vi "Measurement UI.vi"() -> ()   [LabVIEW 2021, in "Crosstalk_Audio ADC_UI.lvlib"]
uses:
  Crosstalk_Audio ADC_UI.lvlib
  shared/controls/PCM Interface Type_Copy.ctl
  <vilib>/PDM Acquisition Toolkit/shared/controls/Digital Edge.ctl
  shared/Audio ADC Shared.lvlib
  <vilib>/PDM Acquisition Toolkit/shared/PDM Shared.lvlib
  shared/controls/Audio ADC Controls.lvlib
panel:
  out "MeasTable":string[][](table)
  in  "MeasGraphs":T1(tab)=enum."Time Domain"
  out "FreqDomainGraph":cluster{"f0":dbl, "df":dbl, "Spectrum":dbl[]}[](graph) caption="AC"
  out "TimeDomainGraph":waveform(dbl)[](graph) caption="AC"
  out "Victim time domain":dbl[](array[numeric])
  out "Victim spectrum":dbl[](array[numeric])
  out "dt":dbl
  out "t0":dbl
  out "df":dbl
  out "f0":dbl
  out "Time domain":dbl[](array[numeric])
  out "Spectrum":dbl[](array[numeric])
  out "Crosstalk":dbl
  out "Channel":string
  in  "Victim channel resource name":string
  in  "Digital capture resource name":string
  in  "Configuration tab":enum32{"Protocol", "Measurement"}(tab)=enum."Measurement"
  in  "Endianness":enum32{"MSB First", "LSB First"}(ring)
  in  "Bit clock edge  sync":enum32{"Rising", "Falling"}(ring)=enum."Falling"
  in  "Frame sync edge for Channel 0":enum32{"Rising", "Falling"}(ring)=enum."Falling"
  in  "Channel count per frame":u32=2
  in  "Channel length":u32=32
  in  "Bit depth":u32=24
  in  "Channel 0 offset":u32=1
  in  "Data Justification":enum32{"Left Justified", "Right Justified"}(ring) caption="Data justification"
  in  "Frame length":u32=64
  in  "Frame sync pulse width":u32=32
  in  "I2S":bool
  in  "LJ":bool
  in  "RJ":bool
  in  "TDM":bool
  in  "Measurement Duration":dbl=0.1 caption="Measurement duration" format="%#_6ps"
  in  "Protocol capture resource name":string(combo) caption="Resource name"
  in  "Analog source resource name":string(combo) caption="Resource name"
  in  "Channel name":string
  in  "Full scale range":dbl=2.825 caption="FULL SCALE RANGE" format="%.3pV"
  in  "Data line":u32
  in  "Sample rate":dbl=192000.0 format="%#.6pHz"
  in  "Measurement settings":string="Measurement Settings"
  in  "Amplitude":dbl=-1.0 format="%#_6pdB"
  in  "Frequency":dbl=1000.0 format="%#_6pHz"
  in  "Victim channel":u32=1
  in  "Interferer channel":u32
  in  "Analog source":string="Analog source"
  in  "Digital capture":string="Digital capture"
  # "Protocols"
  # "PCM data configuration"
  # "Frame sync clock control"
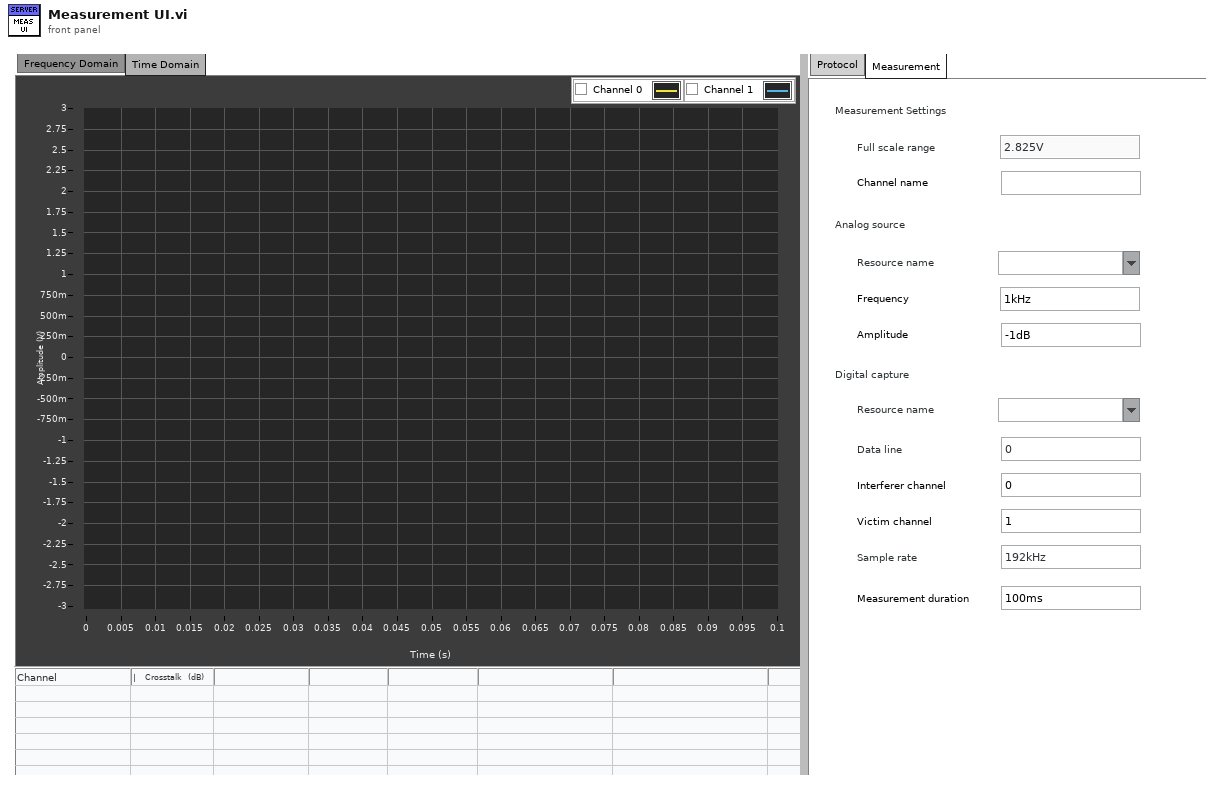
[diagram p1: front panel]
types:
  T1 = enum32{"Frequency Domain", "Time Domain", "Hidden Controls"}
  T2 = typedef "PDM Shared.lvlib/Digital Edge.ctl" = enum8{"Rising", "Falling"}
  T3 = typedef "Audio ADC Controls.lvlib/PCM Interface Type_Copy.ctl" = enum16{"I2S", "Left Justified", "Right Justified", "TDM 4 Channel", "TDM 6 Channel", "TDM 8 Channel", "DSP mode", "DSP mode with 1 bit delay", "PCM Short Frame", "PCM Long Frame"}
  T4 = typedef "PDM Shared.lvlib/PCM Frame Sync Control.ctl" = cluster{"Frame Length":u16, "Frame Sync Pulse Width":u16, "Bit Clock Edge  Sync":T2}
  T5 = typedef "PDM Shared.lvlib/PCM Data Format Configuration.ctl" = cluster{"Frame Sync Edge for Channel 0":T2, "Channel Count Per Frame":u8, "Channel Length":u16, "Bit Depth":u8, "Channel 0 Offset":u16, "Endianness":T6, "Data Justification":T7}
  T6 = typedef "PDM Shared.lvlib/PCM Bit Endianness.ctl" = enum16{"MSB First", "LSB First"}
  T7 = typedef "PDM Shared.lvlib/PCM Data Justification.ctl" = enum16{"Left Justified", "Right Justified"}
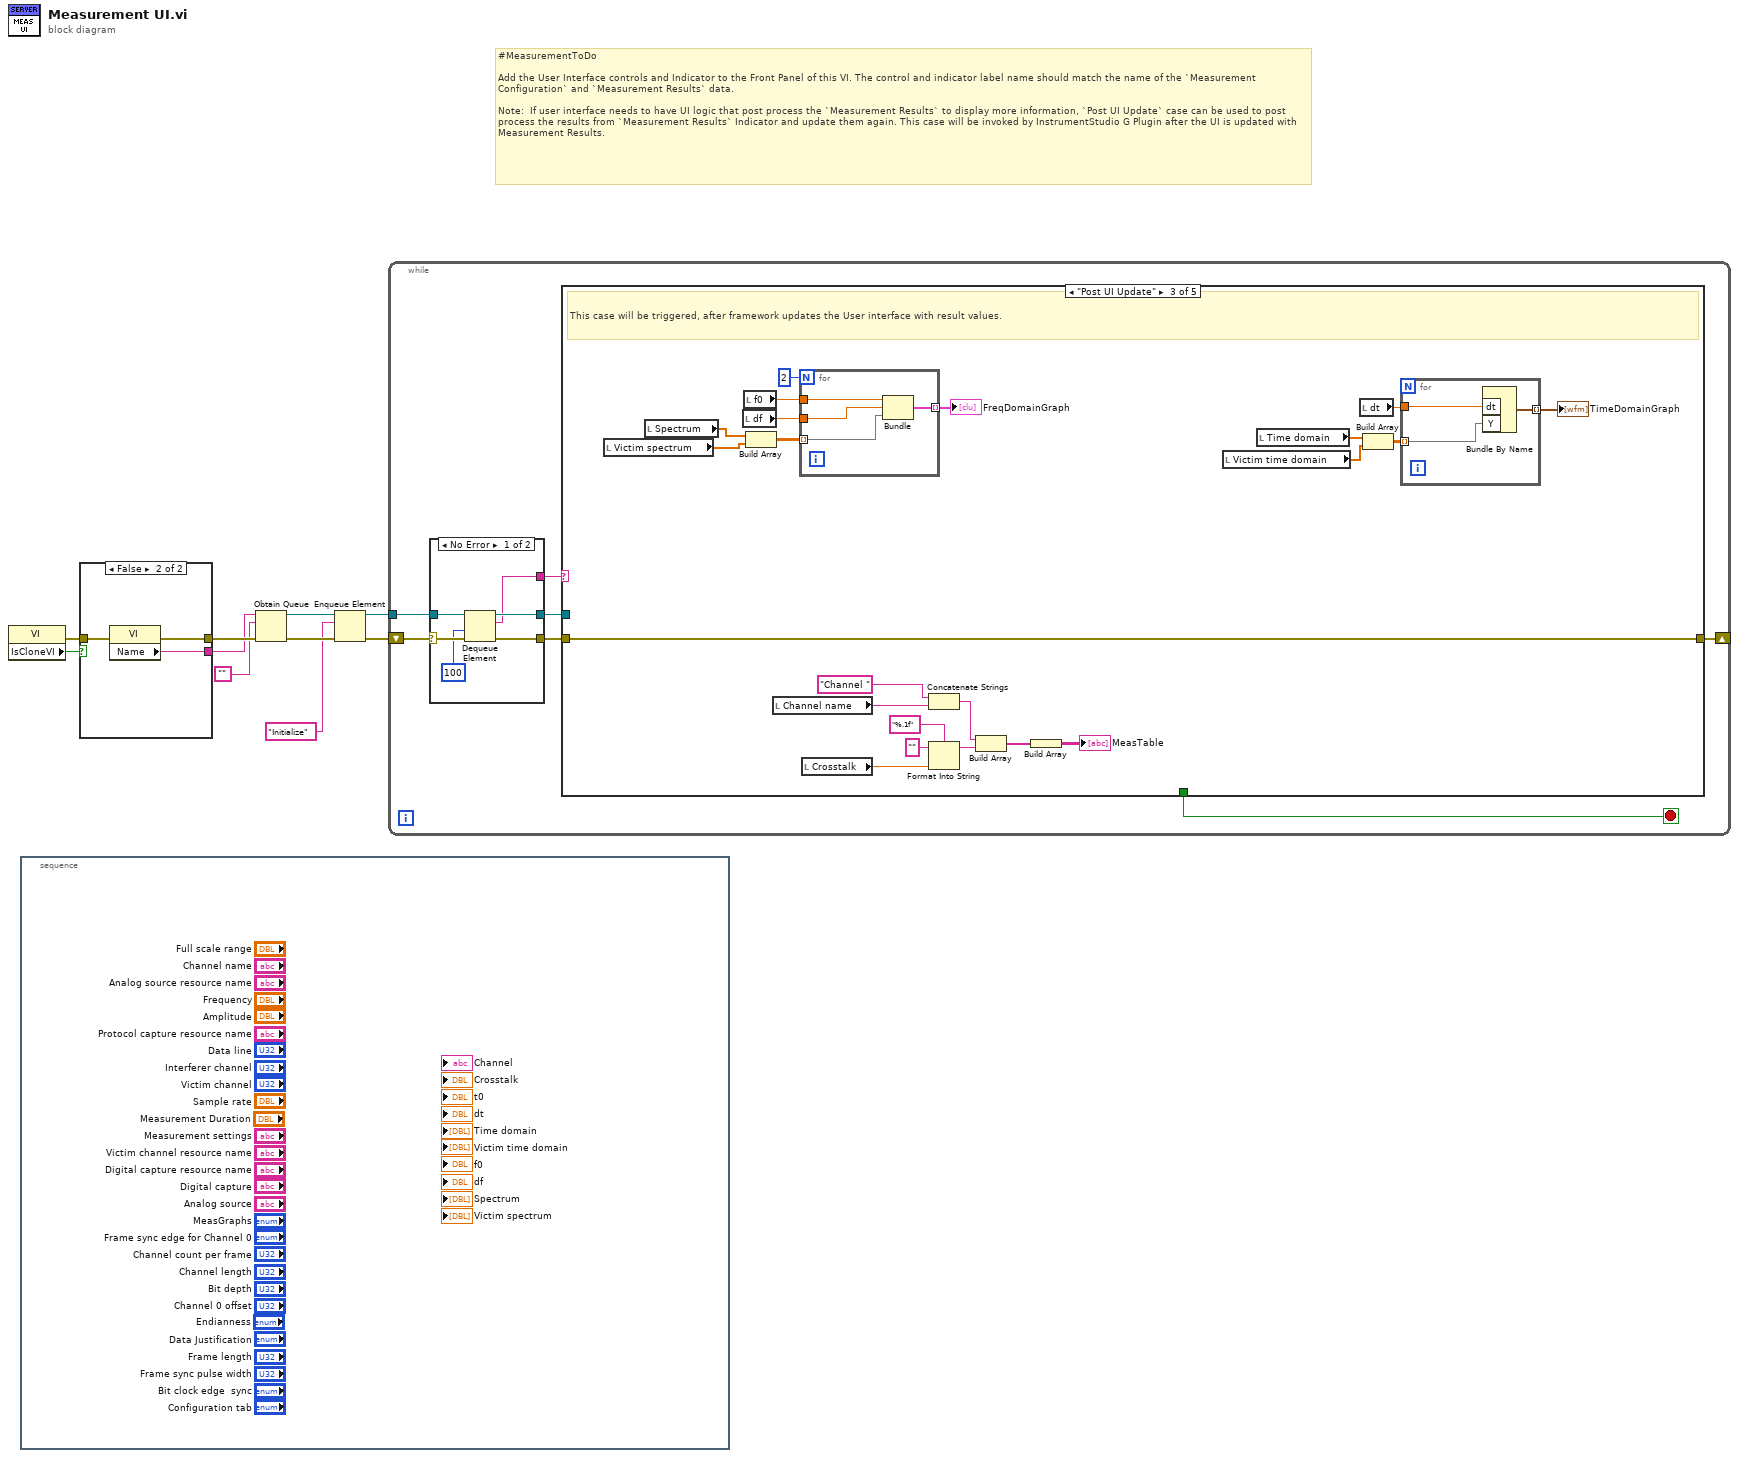
[diagram p0: block diagram]
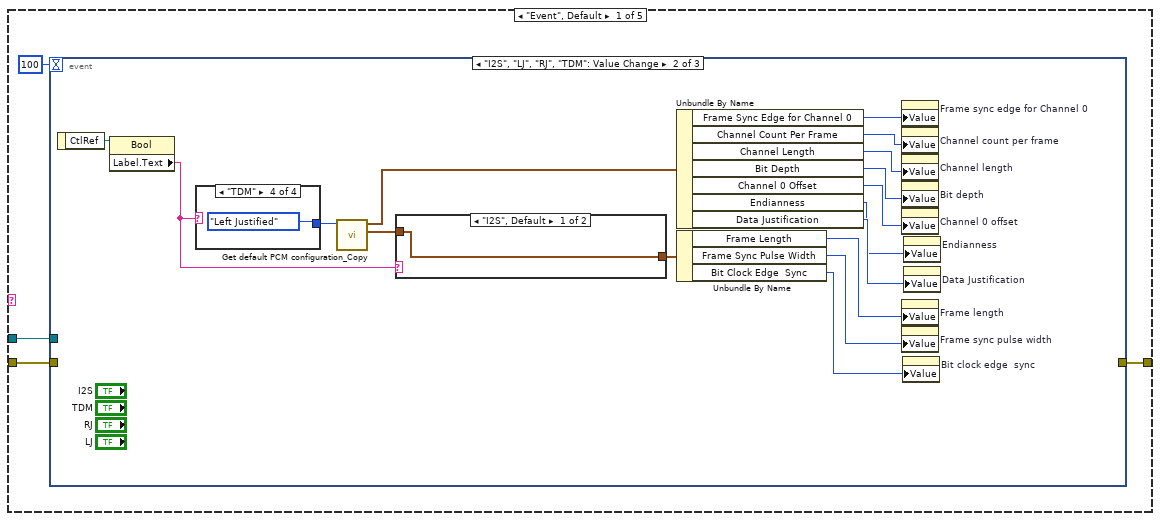
[diagram p2: hidden frame]
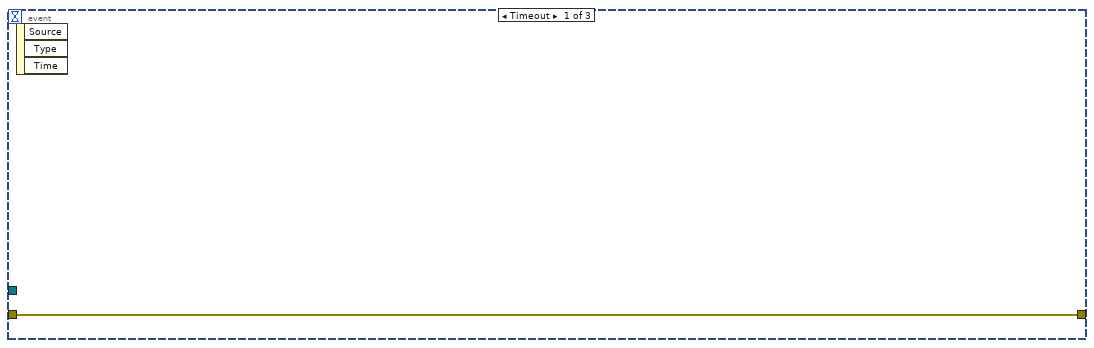
[diagram p3: hidden frame]
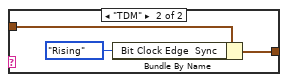
[diagram p4: hidden frame]
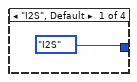
[diagram p5: hidden frame]
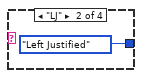
[diagram p6: hidden frame]
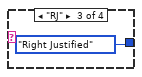
[diagram p7: hidden frame]
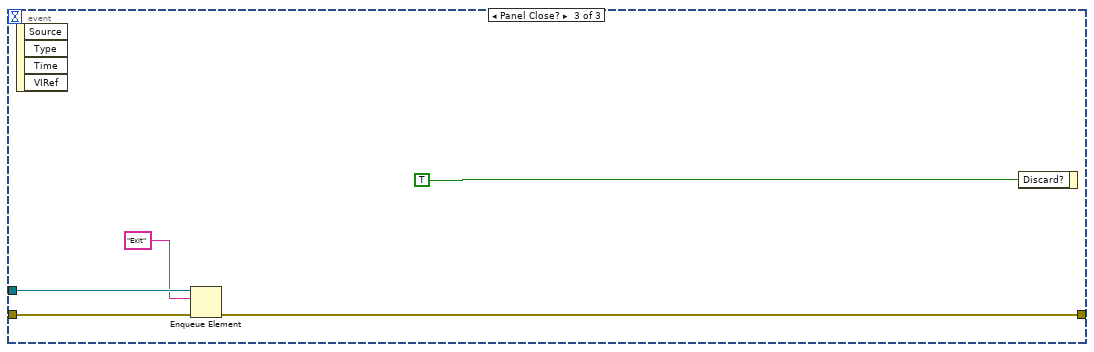
[diagram p8: hidden frame]
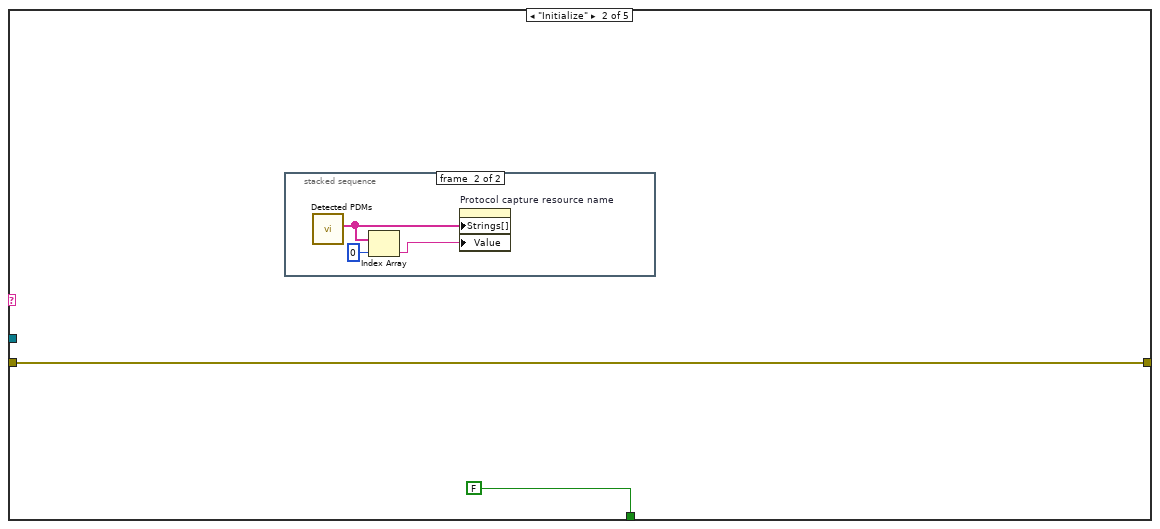
[diagram p9: hidden frame]
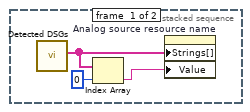
[diagram p10: hidden frame]
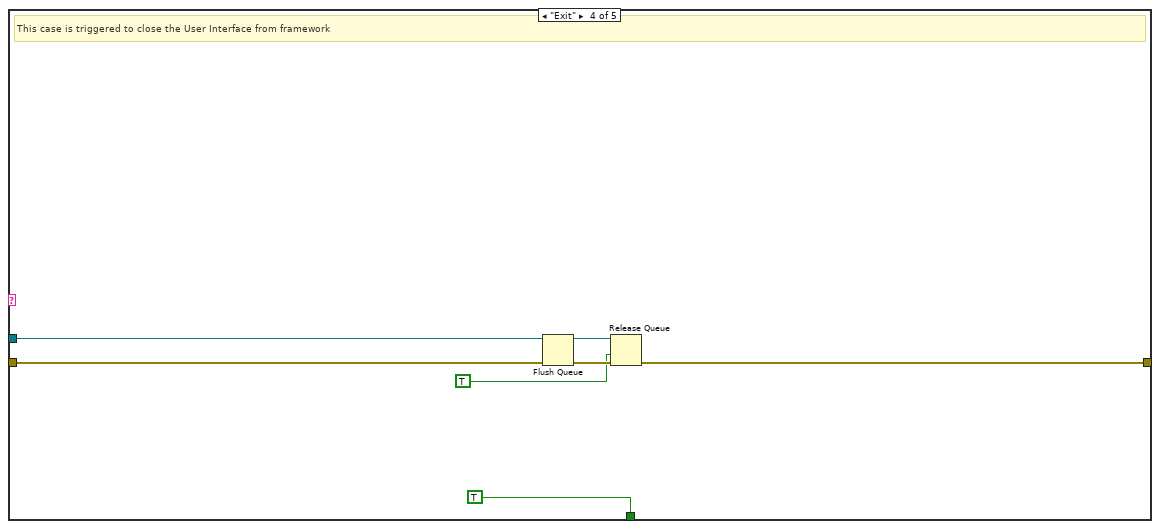
[diagram p11: hidden frame]
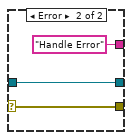
[diagram p13: hidden frame]
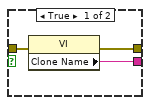
[diagram p14: hidden frame]
diagram:
  # "#MeasurementToDo  \n\nAdd the User Interface controls and Indicator to the Front Panel of this VI. The control and indicator label name should match the name of the `Measurement Configuration` and `Measurement Results` data.\n\nNote:  If user interface needs to have UI logic that post process the `Measurement Results` to display more information, `Post UI Update` case can be used to post process the results from `Measurement Results` Indicator and update them again. This case will be invoked by InstrumentStudio G Plugin after the UI is updated with Measurement Results."
  n1 = property class="VI"() -> (error out=w1:errorcluster, "IsCloneVI"=w2:bool)  [unwired: 2 in, 1 out]
  n2 = stacked-sequence {
    frame #0 {
    }
  }
  n3 = case shown="False" w2 {
    tunnel: [w13 w16] -> w10
    tunnel: [w12 w15] -> w9
    tunnel: w1 -> [w11 w14]
    frame True {
      n4 = property class="VI"(error in=w11) -> (error out=w13:errorcluster, "Clone Name"=w12:string)  [unwired: 1 in, 1 out]
    }
    frame False {
      n5 = property class="VI"(error in=w14) -> (error out=w16:errorcluster, "Name"=w15:string)  [unwired: 1 in, 1 out]
    }
  }
  n6 = Obtain Queue(name (unnamed)=w9, element data type="", error in (no error)=w10) -> (queue out=w6:refnum<queue>, error out=w8:errorcluster)  [unwired: 2 in, 1 out]
  n7 = Enqueue Element(queue=w6, element="Initialize", error in (no error)=w8) -> (queue out=w5:refnum<queue>, error out=w7:errorcluster)  [unwired: 1 in, 1 out]
  n8 = while {
    shift-right: [w18] -> _
    shift-left: w7 -> [w23]
    tunnel: w5 -> [w21]
    stop <- w17 stop-if-true
    n9 = case shown="No Error" w23 {
      selector: w23 -> [w108 w111]
      tunnel: [w107 w111] -> w22
      tunnel: w21 -> [w106 w110]
      tunnel: [w105 w110] -> w20
      tunnel: [w104 "Handle Error"] -> w19
      frame No Error {
        n10 = Dequeue Element(queue=w106, timeout in ms (-1)=100, error in (no error)=w108) -> (queue out=w105:refnum<queue>, element=w104:string, error out=w107:errorcluster)  [unwired: 1 out]
      }
      frame Error {
      }
    }
    n11 = case shown="\"Post UI Update\"" w19 {
      tunnel: w22 -> [w26 w59 w82 w101 w102]
      tunnel: w20 -> [w24 _ _ w99 _]
      tunnel: [w27 w59 w82 w96 w102] -> w18
      tunnel: [_ FALSE _ TRUE _] -> w17
      frame "Event", Default {
        n12 = event shown="[1] \"I2S\", \"LJ\", \"RJ\", \"TDM\": Value Change" {
          selector: _ -> [_ _ _]
          dyn-events: _ -> [_ _ _]
          timeout: 100 -> [_ _ _]
          tunnel: [w28 _ w55] -> w27
          tunnel: w26 -> [w28 _ w56]
          tunnel: w24 -> [_ _ w54]
          event Timeout {
            n13 = event-data() -> ()  [unwired: 1 in, 3 out]
          }
          event "I2S", "LJ", "RJ", "TDM": Value Change {
            n14 = event-data() -> ("CtlRef"=w44:refnum<vi>)  [unwired: 1 in]
            n15 = property class="Bool"(reference=w44) -> ("Label.Text"=w43:string)  [unwired: 1 in, 2 out]
            n16 = case shown="\"TDM\"" w43 {
              tunnel: [PCM_Interface_Type_Copy."I2S" ("PCM Interfaces") PCM_Interface_Type_Copy."Left Justified" ("PCM Interfaces") PCM_Interface_Type_Copy."Right Justified" ("PCM Interfaces") PCM_Interface_Type_Copy."Left Justified" ("PCM Interfaces")] -> w33
              frame "I2S", Default {
              }
              frame "LJ" {
              }
              frame "RJ" {
              }
              frame "TDM" {
              }
            }
            n17 = call "Get default PCM configuration_Copy.vi"("PCM Interfaces"=w33) -> ("Frame Sync Clock Control"=w31:T4, "PCM Data Configuration"=w32:T5)  [unwired: 9 in]
            n18 = case shown="\"I2S\", Default" w43 {
              tunnel: [w45 w47] -> w42
              tunnel: w31 -> [w45 w46]
              frame "I2S", Default {
              }
              frame "TDM" {
                n19 = Bundle By Name(cluster=w46, "Bit Clock Edge  Sync"=Digital_Edge."Rising") -> (w47:T4)
              }
            }
            n20 = Unbundle By Name(w32) -> ("Frame Sync Edge for Channel 0"=w41:T2, "Channel Count Per Frame"=w40:u8, "Channel Length"=w39:u16, "Bit Depth"=w38:u8, "Channel 0 Offset"=w37:u16, "Endianness"=w29:T6, "Data Justification"=w34:T7)
            n21 = Unbundle By Name(w42) -> ("Frame Length"=w36:u16, "Frame Sync Pulse Width"=w35:u16, "Bit Clock Edge  Sync"=w30:T2)
            n22 = property on="Frame sync edge for Channel 0" class="Enum (strict)"("Value"=w41) -> ()  [unwired: 2 in, 2 out]
            n23 = property on="Channel count per frame" class="DigNum (strict)"("Value"=w40) -> ()  [unwired: 2 in, 2 out]
            n24 = property on="Channel length" class="DigNum (strict)"("Value"=w39) -> ()  [unwired: 2 in, 2 out]
            n25 = property on="Bit depth" class="DigNum (strict)"("Value"=w38) -> ()  [unwired: 2 in, 2 out]
            n26 = property on="Channel 0 offset" class="DigNum (strict)"("Value"=w37) -> ()  [unwired: 2 in, 2 out]
            n27 = property on="Frame length" class="DigNum (strict)"("Value"=w36) -> ()  [unwired: 2 in, 2 out]
            n28 = property on="Frame sync pulse width" class="DigNum (strict)"("Value"=w35) -> ()  [unwired: 2 in, 2 out]
            n29 = property on="Bit clock edge  sync" class="Enum (strict)"("Value"=w30) -> ()  [unwired: 2 in, 2 out]
            n30 = property on="Endianness" class="Enum (strict)"("Value"=w29) -> ()  [unwired: 2 in, 2 out]
            n31 = property on="Data Justification" class="Enum (strict)"("Value"=w34) -> ()  [unwired: 2 in, 2 out]
          }
          event Panel Close? {
            n32 = event-data() -> ()  [unwired: 1 in, 4 out]
            n33 = Enqueue Element(queue=w54, element="Exit", error in (no error)=w56) -> (error out=w55:errorcluster)  [unwired: 1 in, 2 out]
            n34 = event-data("Discard?"=TRUE) -> ()  [unwired: 1 in, 1 out]
          }
        }
      }
      frame "Initialize" {
        n35 = stacked-sequence {
          frame #0 {
            n36 = call "Detected DSGs.vi"() -> ("AO channels"=w62:string[])  [unwired: 11 in]
            n37 = Index Array(array=w62, index=0) -> (element=w61:string)
            n38 = property on="Analog source resource name" class="CmbBox"("Strings[]"=w62, "Value"=w61) -> ()  [unwired: 2 in, 2 out]
          }
          frame #1 {
            n39 = call "Detected PDMs.vi"() -> ("PDM devices"=w64:string[])  [unwired: 11 in]
            n40 = Index Array(array=w64, index=0) -> (element=w63:string)
            n41 = property on="Protocol capture resource name" class="CmbBox"("Strings[]"=w64, "Value"=w63) -> ()  [unwired: 2 in, 2 out]
          }
        }
      }
      frame "Post UI Update" {
        # "This case will be triggered, after framework updates the User interface with result values."
        n42 = local read "Victim spectrum"() -> (w74:dbl[])
        n43 = local read "Spectrum"() -> (w75:dbl[])
        n44 = local read "df"() -> (w79:dbl)
        n45 = local read "f0"() -> (w80:dbl)
        n46 = Build Array(w75, w74) -> (w73:dbl[][])
        n47 = local read "Channel name"() -> (w68:string)
        n48 = for {
          N: 2 -> [_]
          tunnel: w80 -> [w94]
          tunnel: w79 -> [w93]
          tunnel: [w92] -> w72 mode=indexing
          tunnel: w73 -> [w91] mode=indexing
          n49 = Bundle("f0"=w94, "df"=w93, w91) -> (w92:cluster{"f0":dbl, "df":dbl, dbl[]})  [unwired: 1 in]
        }
        "FreqDomainGraph" <- w72
        n50 = local read "Crosstalk"() -> (w81:dbl)
        n51 = Concatenate Strings("Channel " ("string"), w68) -> (w67:string)
        n52 = Format Into String(format string="%.1f", initial string="", w81) -> (resulting string=w85:string)  [unwired: 1 in, 1 out]
        n53 = Build Array(w67, w85) -> (w84:string[])
        n54 = Build Array(w84) -> (→"MeasTable":string[][])
        n55 = local read "Victim time domain"() -> (w70:dbl[])
        n56 = local read "Time domain"() -> (w71:dbl[])
        n57 = local read "dt"() -> (w77:dbl)
        n58 = Build Array(w71, w70) -> (w69:dbl[][])
        n59 = for {
          tunnel: [w90] -> w78 mode=indexing
          tunnel: w77 -> [w89]
          tunnel: w69 -> [w88] mode=indexing
          n60 = Bundle By Name("dt"=w89, "Y"=w88) -> (w90:waveform(dbl))  [unwired: 1 in]
        }
        "TimeDomainGraph" <- w78
      }
      frame "Exit" {
        # "This case is triggered to close the User Interface from framework"
        n61 = Flush Queue(queue=w99, error in (no error)=w101) -> (queue out=w98:refnum<queue>, error out=w97:errorcluster)  [unwired: 1 out]
        n62 = Release Queue(queue=w98, force destroy? (F)=TRUE, error in (no error)=w97) -> (error out=w96:errorcluster)  [unwired: 2 out]
      }
      frame "Handle Error" {
      }
    }
  }
